vi "Set Heater.vi"(6 "Channel":i32, 8 "error in (no error)":errorcluster, 10 "Current (A)":dbl, 11 "Instrument.Cryostat in":refnum<class "Instrument.Cryostat.lvclass">) -> (0 "error out":errorcluster, 3 "Instrument.Cryostat out":refnum<class "Instrument.Cryostat.lvclass">)   [LabVIEW 2019, in "Instrument.Cryostat.lvclass"]
uses:
  Instrument.Cryostat.lvclass
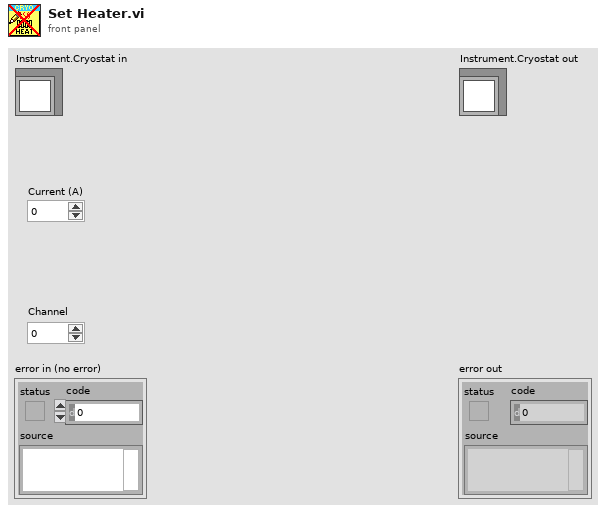
[diagram p1: front panel]
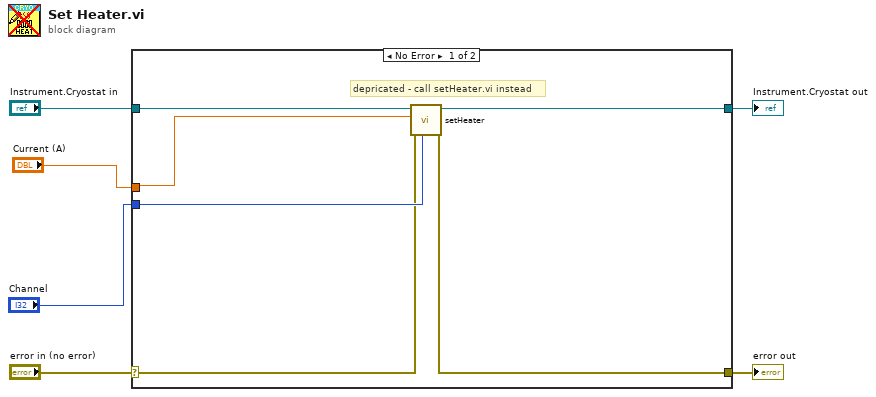
[diagram p0: block diagram]
diagram:
  n1 = case shown="No Error" "error in (no error)" {
    selector: "error in (no error)" -> [w10 w14]
    tunnel: [w9 w14] -> w5
    tunnel: [w8 w13] -> w3
    tunnel: "Instrument.Cryostat in" -> [w7 w13]
    tunnel: "Current (A)" -> [w12 _]
    tunnel: "Channel" -> [w11 _]
    frame No Error {
      # "depricated - call setHeater.vi instead"
      n2 = call-dynamic "setHeater.vi"("Channel"=w11, "error in (no error)"=w10, "Current (A)"=w12, "Instrument.Cryostat in"=w7) -> ("error out"=w9:errorcluster, "Instrument.Cryostat out"=w8:refnum<class "Instrument.Cryostat.lvclass">)  [unwired: 6 in]
    }
    frame Error {
    }
  }
  "error out" <- w5
  "Instrument.Cryostat out" <- w3
